vi "Handle Command.vi"(8 "error in (no error)":errorcluster, 9 "Value":bool, 11 "SequencedValves in":refnum<class "DelayControl.lvclass">) -> (0 "error out":errorcluster, 3 "SequencedValves out":refnum<class "DelayControl.lvclass">)   [LabVIEW 2020, in "VolatusControl.lvlib" / "DelayControl.lvclass"]
uses:
  DelayControl.lvclass
  DelayControl.lvclass/DelayControl.ctl
  State.ctl
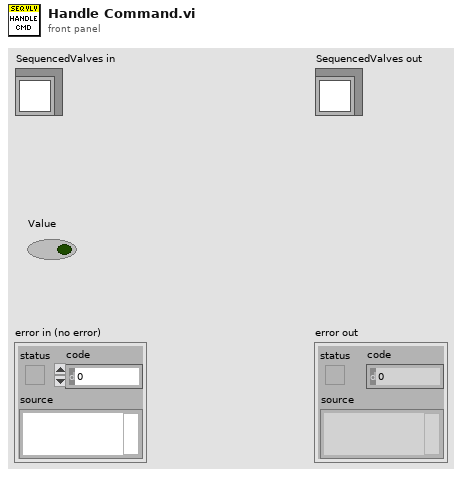
[diagram p1: front panel]
types:
  T1 = typedef "VolatusControl.lvlib/DelayControl.lvclass/State.ctl" = enum16{"Idle", "Start", "Delay"}
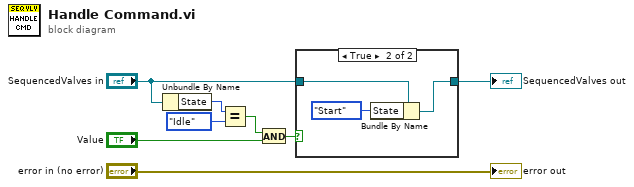
[diagram p0: block diagram]
diagram:
  n1 = Unbundle By Name("SequencedValves in") -> ("State"=w5:T1)
  n2 = Equal?(x=w5, y=State."Idle") -> (x = y?=w2:bool)
  n3 = And(x=w2, y="Value") -> (x .and. y?=w3:bool)
  n4 = case shown="True" w3 {
    tunnel: "SequencedValves in" -> [w9 w12]
    tunnel: [w9 w10] -> w1
    frame False {
    }
    frame True {
      n5 = Bundle By Name(cluster=w12, "State"=State."Start") -> (w10:refnum<class "DelayControl.lvclass">)
    }
  }
  "SequencedValves out" <- w1
  "error out" <- "error in (no error)"
